vi "initializeCounters.vi"(5 "Sample Time":dbl=0.02 format="%0.2f") -> (0 "error out":errorcluster, 2 "task out":refnum<k21>)   [LabVIEW 2012]
uses:
  <vilib>/DAQmx/create/channels.llb/DAQmx Create Channel (CO-Pulse Generation-Frequency).vi
  <vilib>/DAQmx/configure/timing.llb/DAQmx Timing (Implicit).vi
  <vilib>/DAQmx/create/channels.llb/DAQmx Create Channel (CI-Count Edges).vi
  <vilib>/DAQmx/configure/timing.llb/DAQmx Timing (Sample Clock).vi
  <resource>/objmgr/daqmx.rc
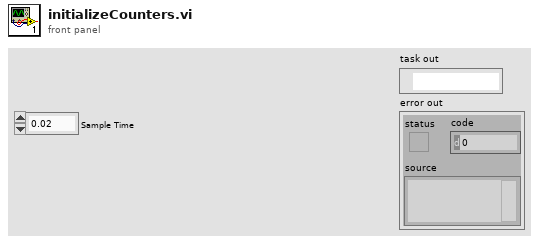
[diagram p1: front panel]
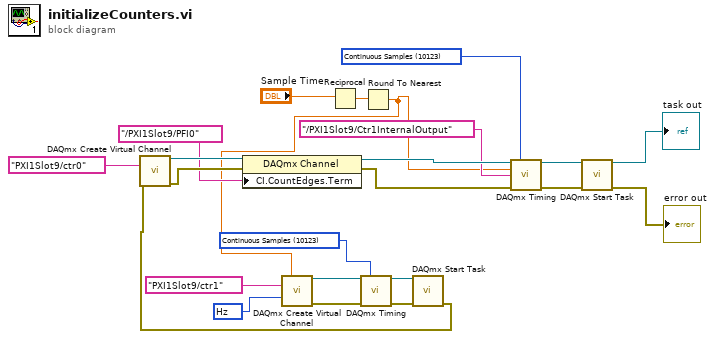
[diagram p0: block diagram]
diagram:
  w6 = 10123 items=["Finite Samples"=10178, "Continuous Samples"=10123, "Hardware Timed Single Point"=12522] ("sample mode")
  w12 = 10373 items=["Hz"=10373] ("units")
  w15 = 10123 items=["Finite Samples"=10178, "Continuous Samples"=10123, "Hardware Timed Single Point"=12522] ("sample mode")
  n1 = Reciprocal(x="Sample Time") -> (1/x=w4:dbl)
  n2 = Round To Nearest(number=w4) -> (nearest integer value=w3:dbl)
  n3 = call-poly <vilib>:"DAQmx Create Virtual Channel.vi"("frequency"=w3, "counter"=tag "PXI1Slot9/ctr1", "units"=w12) -> ("task out"=w10:refnum<k21>, "error out"=w9:errorcluster)  [unwired: 11 in]
  n4 = call-poly <vilib>:"DAQmx Timing.vi"("task/channels in"=w10, "sample mode"=w6, "error in"=w9) -> ("task out"=w8:refnum<k21>, "error out"=w7:errorcluster)  [unwired: 11 in]
  n5 = call <vilib>:"DAQmx Start Task.vi"("task/channels in"=w8, "error in"=w7) -> ("error out"=w13:errorcluster)  [unwired: 12 in, 1 out]
  n6 = call-poly <vilib>:"DAQmx Create Virtual Channel.vi"("counter"=tag "PXI1Slot9/ctr0", "error in"=w13) -> ("task out"=w18:refnum<k21>, "error out"=w17:errorcluster)  [unwired: 12 in]
  n7 = property class="DAQmx Channel"(reference=w18, error in=w17, "CI.CountEdges.Term"=tag "/PXI1Slot9/PFI0") -> (reference out=w20:refnum<k21>, error out=w19:errorcluster)
  n8 = call-poly <vilib>:"DAQmx Timing.vi"("task/channels in"=w20, "sample mode"=w15, "rate"=w3, "source"=tag "/PXI1Slot9/Ctr1InternalOutput", "error in"=w19) -> ("task out"=w22:refnum<k21>, "error out"=w21:errorcluster)  [unwired: 9 in]
  n9 = call <vilib>:"DAQmx Start Task.vi"("task/channels in"=w22, "error in"=w21) -> ("task out"=→"task out":refnum<k21>, "error out"=→"error out":errorcluster)  [unwired: 12 in]
